vi "List Sweep.vi"(7 "Sweep Points Value":string, 8 "error in (no error)":errorcluster, 9 "Sweep Mode (T: Sequence)":bool=TRUE, 10 "List Function (0: Frequency)":u32(slide) max=4 step=1, 11 "VISA resource name":refnum<visa-resource-name>) -> (0 "error out":errorcluster, 3 "VISA resource name out":refnum<visa-resource-name>)   [LabVIEW 2015, in "Agilent 428X Series.lvlib"]
doc: "This VI sets the List Sweep measurement function, including the sweep point settings and the Sweep Mode."
uses:
  Agilent 428X Series.lvlib
panel:
  # "Sequence\nStepped"
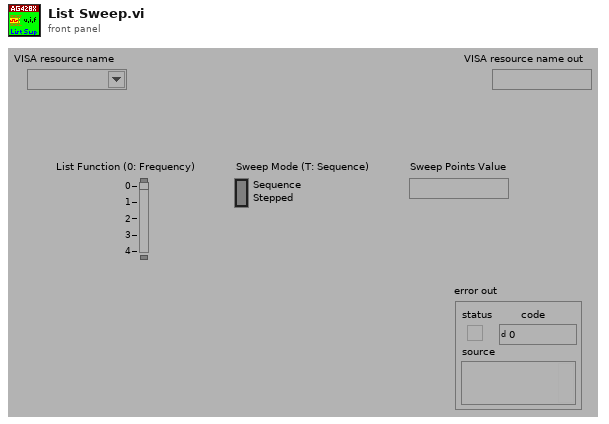
[diagram p1: front panel]
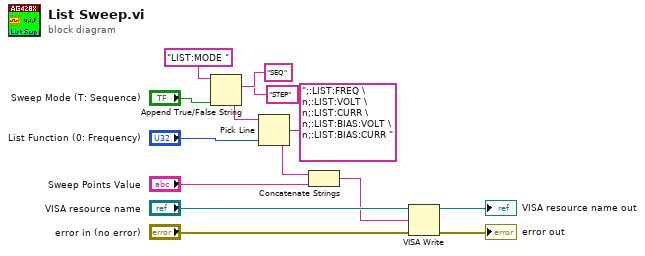
[diagram p0: block diagram]
diagram:
  n1 = Append True/False String(1:"Sweep Mode (T: Sequence)", 2:"STEP" ("false string"), 3:"SEQ" ("true string"), 4:"LIST:MODE " ("string (\"\")")) -> (0:w5:string)
  n2 = Pick Line(string ("")=w5, multi-line string=";:LIST:FREQ \n;:LIST:VOLT \n;:LIST:CURR \n;:LIST:BIAS:VOLT \n;:LIST:BIAS:CURR ", line index="List Function (0: Frequency)") -> (output string=w2:string)
  n3 = Concatenate Strings(w2, "Sweep Points Value") -> (w1:string)
  n4 = VISA Write(VISA resource name="VISA resource name", write buffer=w1, error in (no error)="error in (no error)") -> (VISA resource name out=→"VISA resource name out":refnum<visa-resource-name>, error out=→"error out":errorcluster)  [unwired: 1 out]
